vi "Target LRN Controller.vi"(6 "Learning Gains":T1={"KL"=15.0, "Beta"=0.97, "D"=18}, 7 "Error":dbl, 8 "Phase":dbl, 9 "HS":bool, 11 "Active?":bool) -> (3 "UFF":dbl)   [LabVIEW 2018, in "COBRA Iterative Learning Control Library.lvlib"]
uses:
  COBRA Iterative Learning Control Library.lvlib
  Target Learning Gains.ctl
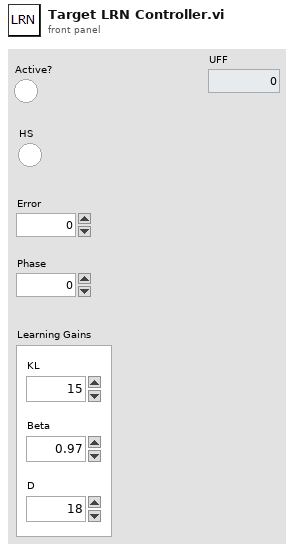
[diagram p1: front panel]
types:
  T1 = typedef "COBRA Iterative Learning Control Library.lvlib/Target Learning Gains.ctl" = cluster{"KL":dbl, "Beta":dbl, "D":i32}
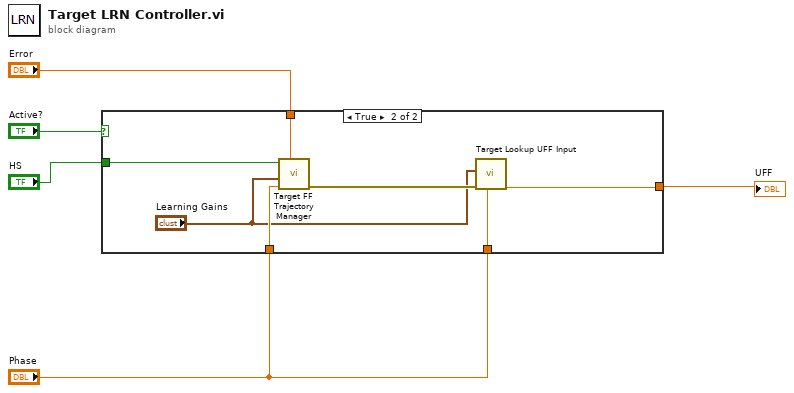
[diagram p0: block diagram]
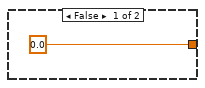
[diagram p2: hidden frame]
diagram:
  n1 = case shown="True" "Active?" {
    tunnel: [0.0 ("y") w8] -> w1
    tunnel: "HS" -> [_ w13]
    tunnel: "Phase" -> [_ w10]
    tunnel: "Phase" -> [_ w12]
    tunnel: "Error" -> [_ w11]
    frame False {
    }
    frame True {
      n2 = call "Target FF Trajectory Manager.vi"("Error"=w11, "Phase"=w12, "Learning Gains"="Learning Gains", "HS"=w13) -> ("Error Out"=w9:errorcluster)  [unwired: 7 in]
      n3 = call "Target Lookup UFF Input.vi"("Phase"=w10, "Error In"=w9, "Learning Gains"="Learning Gains") -> ("UFF"=w8:dbl)  [unwired: 8 in]
    }
  }
  "UFF" <- w1
